vi "System - CalScope and Trends.vi"() -> ()   [LabVIEW 2015, in "ECS-Host.lvlib"]
uses:
  ECS-Host.lvlib
  <vilib>/addons/Software Calibration Management/XControls/CalScope.xctl
  <vilib>/addons/Software Calibration Management/XControls/CalTrend.xctl
panel:
  in  "CalTrend":cluster{"Data":dbl}(xcontrol)
  in  "CalScope":T1[](xcontrol)
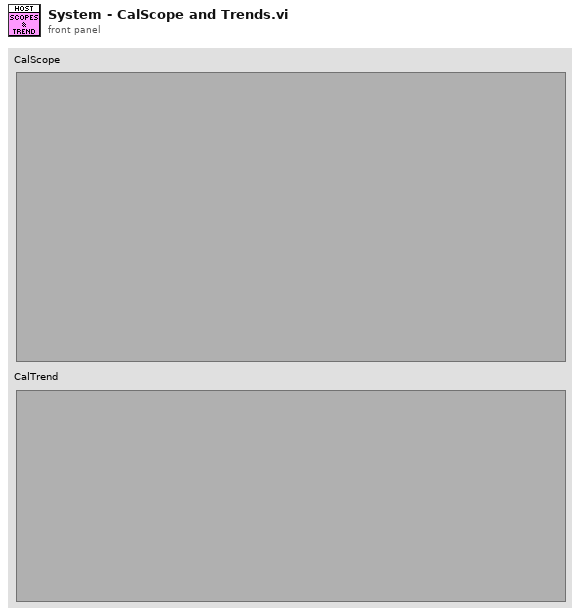
[diagram p1: front panel]
types:
  T1 = typedef "CalScope.xctl/CalScope - Data Set.ctl" = cluster{"ScopeData":sgl[]}
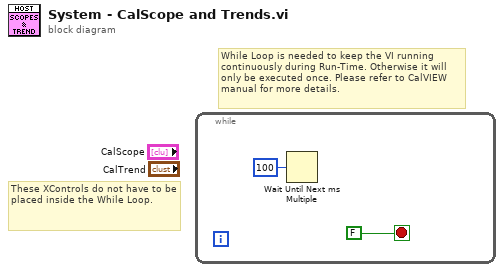
[diagram p0: block diagram]
diagram:
  # "While Loop is needed to keep the VI running\ncontinuously during Run-Time. Otherwise it will only be executed once. Please refer to CalVIEW manual for more details."
  # "These XControls do not have to be placed inside the While Loop."
  n1 = while {
    stop <- FALSE stop-if-true
    n2 = Wait Until Next ms Multiple(millisecond multiple=u32 100) -> ()  [unwired: 1 out]
  }
